vi "test_python_labview_intigration_1.vi"() -> ()   [LabVIEW 2020]
panel:
  out "return value":i32[](array[numeric])
  out "appended path":path
  in  "error in (no error)":errorcluster
  in  "goal y":dbl
  in  "goal x":dbl
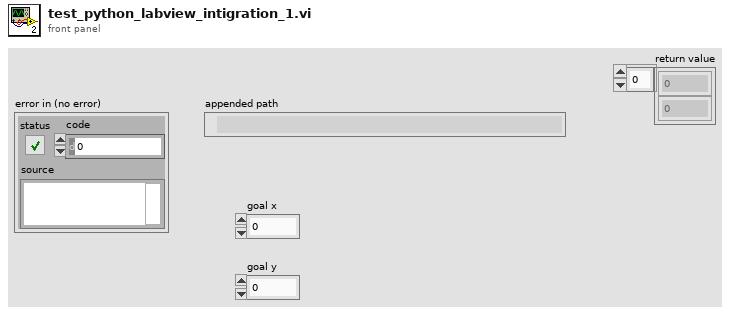
[diagram p1: front panel]
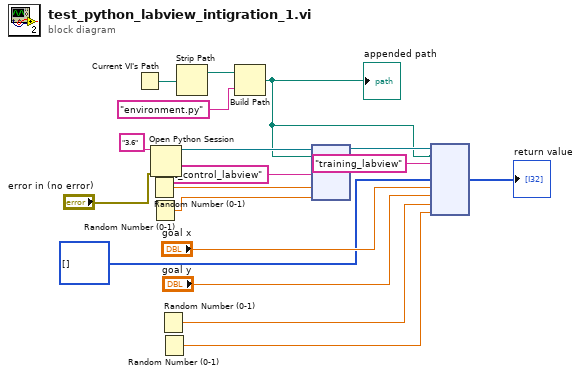
[diagram p0: block diagram]
diagram:
  n1 = Current VI's Path() -> (path=w13:path)
  n2 = Random Number (0-1)() -> (number: 0 to 1=w8:dbl)
  n3 = Random Number (0-1)() -> (number: 0 to 1=w7:dbl)
  n4 = Open Python Session(python version="3.6" ("Python version"), 3:"error in (no error)") -> (session out=w17:refnum<k35>)  [unwired: 1 in, 1 out]
  n5 = Random Number (0-1)() -> (number: 0 to 1=w2:dbl)
  n6 = Random Number (0-1)() -> (number: 0 to 1=w1:dbl)
  n7 = Strip Path(path=w13) -> (stripped path=w12:path)  [unwired: 1 out]
  n8 = Build Path(base path=w12, name or relative path="environment.py") -> (appended path=w10:path)
  "appended path" <- w10
  n9 = node(w17, w10, "init_control_labview" ("function name"), w8, w7) -> (w16:refnum<k35>)  [unwired: 5 in, 3 out]
  n10 = node(w16, w10, "training_labview" ("function name"), i32[] [], "goal x", "goal y", w2, w1) -> (→"return value":i32[])  [unwired: 5 in, 4 out]
